vi "ITX Folder to TDMS.vi"(8 "error in (no error)":errorcluster, 11 "Folder Path":path) -> (0 "error out":errorcluster)   [LabVIEW 2016, in "Conversion.lvclass"]
uses:
  Conversion.lvclass
  Data/Data.lvclass
panel:
  in  "stop":bool
  in  "Additional Notes?":string
  in  "Single File?":bool
  out "Elapsed Time (s)":dbl
  out "Numeric":i32
  # "T = Create 1 TDMS file for the entire folder\nF = Create 1 TDMS file for each ITX file"
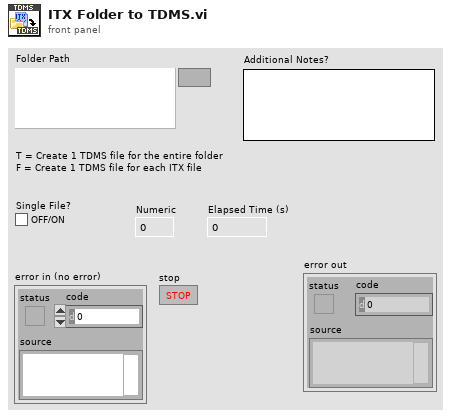
[diagram p1: front panel]
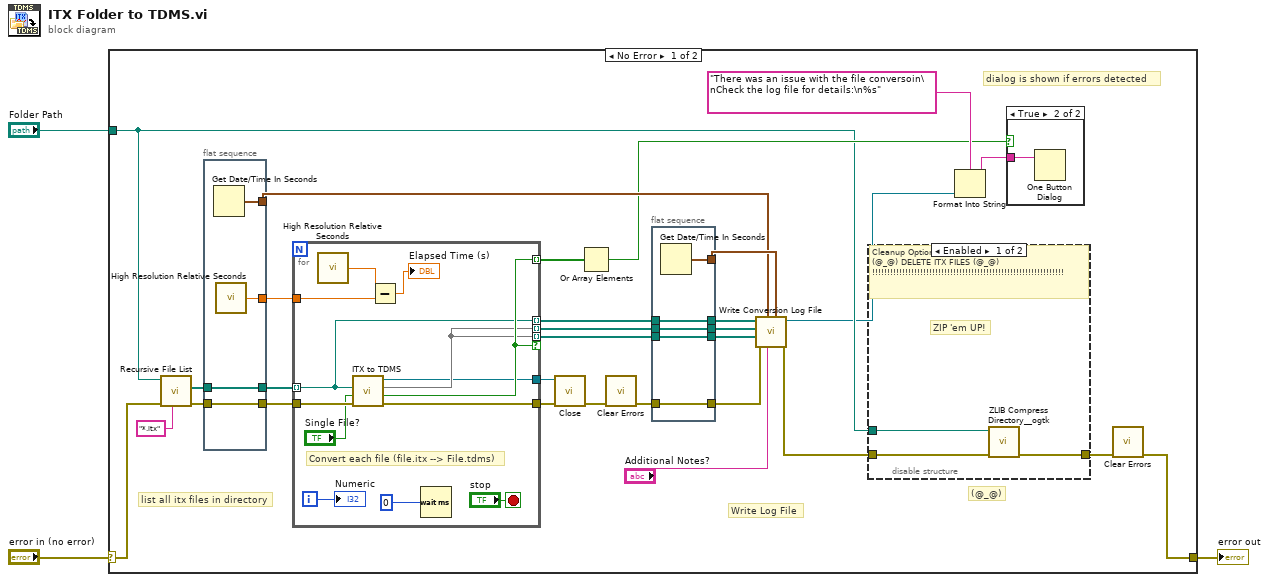
[diagram p0: block diagram]
diagram:
  n1 = case shown="No Error" "error in (no error)" {
    selector: "error in (no error)" -> [w32 w61]
    tunnel: [w8 w61] -> w2
    tunnel: "Folder Path" -> [w11 _]
    frame No Error {
      # "(@_@)"
      # "dialog is shown if errors detected"
      # "list all itx files in directory"
      # "Write Log File"
      n2 = call <vilib>:"Recursive File List.vi"("pattern"="*.itx", "error in (no error)"=w32, "Folder Path"=w11) -> ("error out"=w28:errorcluster, "All Files in Dir"=w27:path[])  [unwired: 4 in, 3 out]
      n3 = flat-sequence {
        tunnel: [w42] -> w31
        tunnel: [w41] -> w29
        tunnel: w28 -> [w41]
        tunnel: w27 -> [w40]
        tunnel: [w40] -> w26
        tunnel: [w39] -> w15
        frame #0 {
          n4 = Get Date/Time In Seconds() -> (seconds since 1Jan1904=w39:timestamp)
          n5 = call <vilib>:"High Resolution Relative Seconds.vi"() -> ("relative seconds"=w42:dbl)
        }
      }
      n6 = for {
        tunnel: w26 -> [w48] mode=indexing
        tunnel: w29 -> [w60]
        tunnel: [w59] -> w5
        tunnel: w31 -> [w56]
        tunnel: [w51] -> w22 mode=indexing if=w52
        tunnel: [w51] -> w24 mode=indexing
        tunnel: [w48] -> w25 mode=indexing
        tunnel: [w52] -> w30 mode=indexing
        tunnel: [w50] -> w6
        i -> [w58]
        stop <- "stop" stop-if-true
        # "Convert each file (file.itx --> File.tdms)"
        n7 = call <vilib>:"High Resolution Relative Seconds.vi"() -> ("relative seconds"=w57:dbl)
        n8 = call "ITX to TDMS.vi"("error in (no error)"=w60, "Single File? [T]"="Single File?", "Path"=w48) -> ("error out"=w59:errorcluster, "Not Equal?"=w52:bool, 2:w51, "Conversion.lvclass out"=w50:refnum<class "Conversion.lvclass">)  [unwired: 5 in]
        n9 = Subtract(x=w57, y=w56) -> (x-y=→"Elapsed Time (s)":dbl)
        n10 = Wait (ms)(milliseconds to wait=u32 0) -> ()  [unwired: 1 out]
        "Numeric" <- w58
      }
      n11 = call-dynamic "Close.vi"("error in (no error)"=w5, "Data in"=w6) -> ("error out"=w4:errorcluster)  [unwired: 8 in, 1 out]
      n12 = Or Array Elements(Boolean array=w30) -> (logical OR=w12:bool)
      n13 = call <vilib>:"Clear Errors.vi"("error in (no error)"=w4) -> ("error out"=w9:errorcluster)  [unwired: 5 in, 1 out]
      n14 = flat-sequence {
        tunnel: w25 -> [w37]
        tunnel: [w38] -> w17
        tunnel: w24 -> [w38]
        tunnel: [w37] -> w18
        tunnel: [w36] -> w23
        tunnel: w22 -> [w36]
        tunnel: w9 -> [w35]
        tunnel: [w35] -> w13
        tunnel: [w34] -> w21
        frame #0 {
          n15 = Get Date/Time In Seconds() -> (seconds since 1Jan1904=w34:timestamp)
        }
      }
      n16 = call "Write Conversion Log File.vi"(5:w21, 6:"Additional Notes?", 7:w15, "error in (no error)"=w13, 9:w23, "Additional Notes?"=w17, "Conversion.lvclass"=w18) -> ("error out"=w14:errorcluster, "Conversion.lvclass out"=w10:refnum<class "Conversion.lvclass">)  [unwired: 2 in, 1 out]
      n17 = disable-structure shown="Enabled" {
        disable-tunnel: w14 -> [w44 w46]
        disable-tunnel: [w43 w46] -> w16
        disable-tunnel: w11 -> [w45 _]
        frame Enabled {
          # "ZIP 'em UP!"
          # "Cleanup Option:\n(@_@) DELETE ITX FILES (@_@)\n!!!!!!!!!!!!!!!!!!!!!!!!!!!!!!!!!!!!!!!!!!!!!!!!!!!!!!!!!!!!!!!!"
          n18 = call <userlib>:"ZLIB Compress Directory__ogtk.vi"("error in (no error)"=w44, "root directory (file dialog)"=w45) -> ("error out"=w43:errorcluster)  [unwired: 7 in, 2 out]
        }
        frame Disabled {
        }
      }
      n19 = Format Into String(format string="There was an issue with the file conversoin\nCheck the log file for details:\n%s", w10) -> (resulting string=w20:string)  [unwired: 2 in, 1 out]
      n20 = case shown="True" w12 {
        tunnel: w20 -> [_ w47]
        frame False {
        }
        frame True {
          n21 = One Button Dialog(message=w47) -> ()  [unwired: 1 in, 1 out]
        }
      }
      n22 = call <vilib>:"Clear Errors.vi"("error in (no error)"=w16) -> ("error out"=w8:errorcluster)  [unwired: 5 in, 1 out]
    }
    frame Error {
    }
  }
  "error out" <- w2
